vi "垫片有无显示ROI - 副本.vi"(0 "原始图像 IN":T4(plugin-control), 1 "Font, Size & Style":T1={"Desired Font (Application)"=enum."Application Font", "[User-specified Font]"={"Font Name"="", "Size"=100, "Strikeout?"=FALSE, "Italic?"=FALSE, "Underline?"=FALSE, "Outline?"=FALSE, "Shadow?"=FALSE, "Bold?"=TRUE, "Rotation Angle"=0.0}, "Horizontal Alignment"=0, "Vertical Alignment"=0} {"Horizontal Alignment" items=["Left", "Center", "Right"]; "Vertical Alignment" items=["Bottom", "Top", "Baseline"]}, 3 "Center X":i32, 5 "ROI Descriptor":T3 {"Contours"."Type" items=["No Selection", "Point", "Line", "Rectangle", "Oval", "Polygon", "Freehand Region", "Annulus", "Unused2", "Unused3", "Broken Line", "Freehand Line", "Rotated Rectangle"]}, 9 "黑像素阀值判定个数":dbl, 11 "error in (no error)":errorcluster caption="错误输入（无错误）", 12 "黑像个数":dbl, 13 "Center Y":i32) -> (4 "原始图像 OUT":T4(plugin-control), 6 "铜片有/无":bool, 10 "异常":bool, 15 "error out":errorcluster caption="错误输出")   [LabVIEW 2017]
panel:
  out "Annulus":T2 {"End Angle" min=-90.0 max=90.0 step=1.0 format="%.2f"; "Start Angle" min=-90.0 max=90.0 step=1.0 format="%.2f"; "Center X" scale=0.0..1024.0}
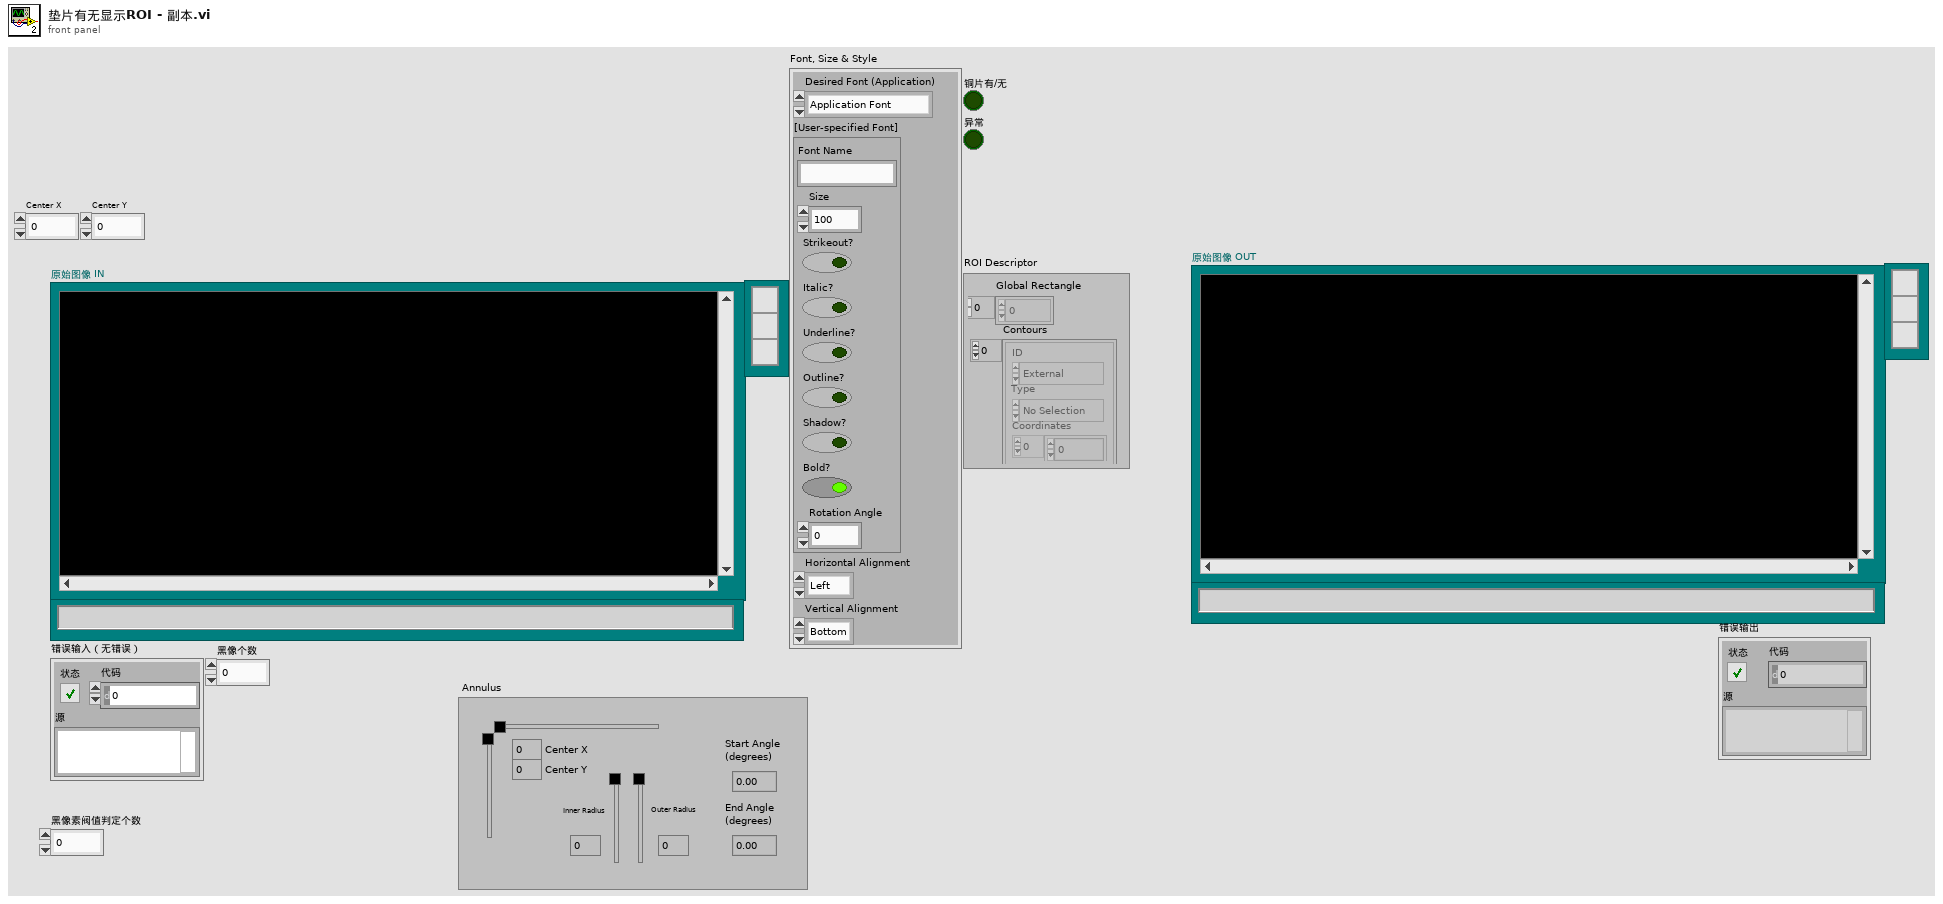
[diagram p1: front panel]
types:
  T1 = cluster{"Desired Font (Application)":enum16{"User-specified Font", "Application Font", "System Font", "Dialog Font"}, "[User-specified Font]":cluster{"Font Name":string, "Size":i16, "Strikeout?":bool, "Italic?":bool, "Underline?":bool, "Outline?":bool, "Shadow?":bool, "Bold?":bool, "Rotation Angle":dbl}, "Horizontal Alignment":i16, "Vertical Alignment":i16}
  T2 = typedef "IMAQ Circle" = cluster{"Center X":i32, "Center Y":i32, "Inner Radius":i32, "Outer Radius":i32, "Start Angle":dbl, "End Angle":dbl}
  T3 = typedef "ROI Descriptor" = cluster{"Global Rectangle":i32[], "Contours":cluster{"ID":enum32{"External", "Internal"}, "Type":u32, "Coordinates":i32[]}[]}
  T4 = typedef "IMAQ Image.ctl" = refnum<image>
  T5 = cluster{"Left":i32, "Top":i32, "rigte":i32, "bottom 3":i32}
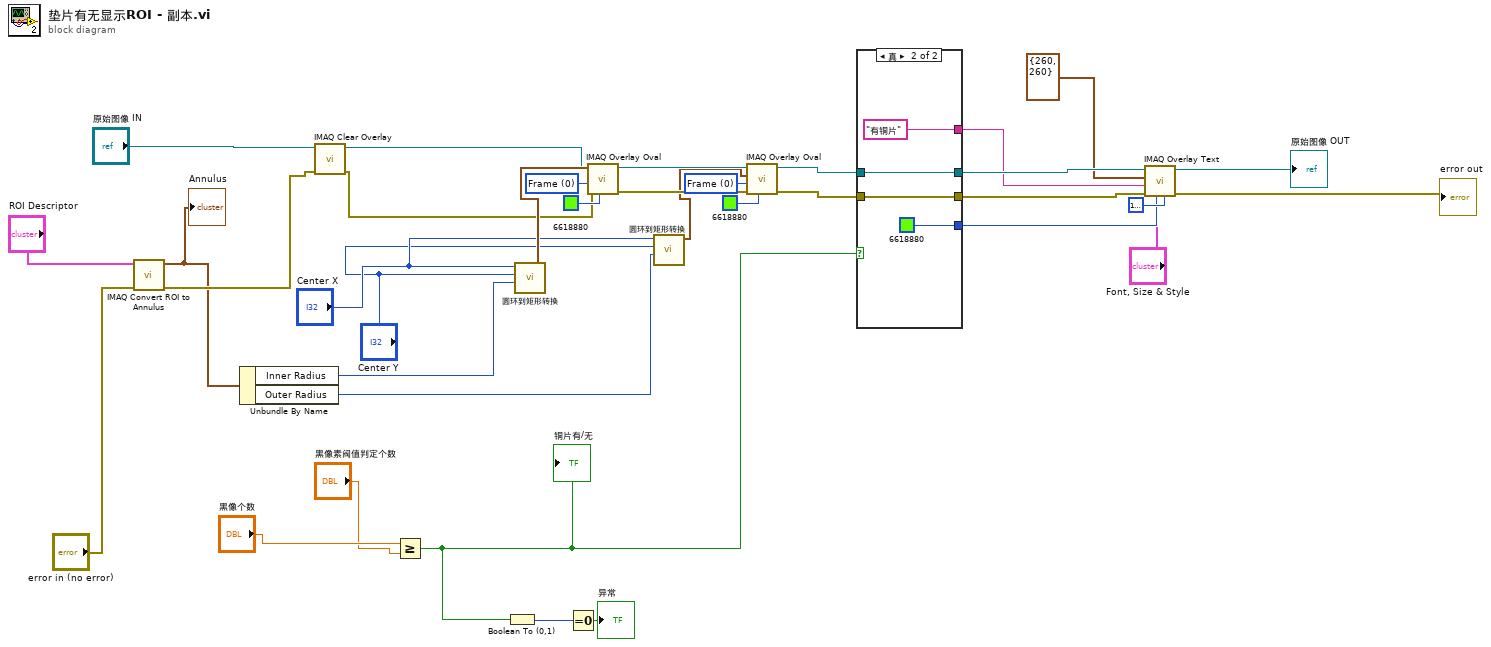
[diagram p0: block diagram]
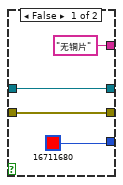
[diagram p2: hidden frame]
diagram:
  w32 = u32 0 items=["Frame", "Fill"] ("Drawing Mode (Frame)")
  w35 = u32 0 items=["Frame", "Fill"] ("Drawing Mode (Frame)")
  n1 = call "IMAQ Convert ROI to Annulus"("error in (no error)"="error in (no error)", "ROI Descriptor"="ROI Descriptor") -> ("error out"=w10:errorcluster, "Annulus"=w2:T2)  [unwired: 7 in]
  "Annulus" <- w2
  n2 = Unbundle By Name(w2) -> ("Inner Radius"=w27:i32, "Outer Radius"=w25:i32)
  n3 = call "IMAQ Clear Overlay"("error in (no error)"=w10, "Image"="原始图像 IN") -> ("error out"=w9:errorcluster, "Image Out"=w11:T4)  [unwired: 8 in]
  n4 = Greater Or Equal?(x="黑像个数", y="黑像素阀值判定个数") -> (x >= y?=w8:bool)
  "铜片有/无" <- w8
  n5 = Boolean To (0,1)(Boolean=w8) -> (0, 1=w7:i16)
  n6 = call "圆环到矩形转换.vi"("Radius"=w27, "CenerY"="Center Y", "CenerX"="Center X") -> ("Bounding Rectangle out"=w28:T5)  [unwired: 8 in]
  n7 = Equal To 0?(x=w7) -> (x = 0?=→"异常":bool)
  n8 = call "IMAQ Overlay Oval"("Color"=u32 6618880, "error in (no error)"=w9, "Drawing Mode (Frame)"=w35, "Bounding Rectangle"=w28, "Image"=w11) -> ("error out"=w33:errorcluster, "Image Out"=w34:T4)  [unwired: 5 in]
  n9 = call "圆环到矩形转换.vi"("Radius"=w25, "CenerY"="Center Y", "CenerX"="Center X") -> ("Bounding Rectangle out"=w26:T5)  [unwired: 8 in]
  n10 = call "IMAQ Overlay Oval"("Color"=u32 6618880, "error in (no error)"=w33, "Drawing Mode (Frame)"=w32, "Bounding Rectangle"=w26, "Image"=w34) -> ("error out"=w21:errorcluster, "Image Out"=w22:T4)  [unwired: 5 in]
  n11 = case shown="真" w8 {
    tunnel: w22 -> [w39 w43]
    tunnel: w21 -> [w38 w42]
    tunnel: [w39 w43] -> w20
    tunnel: [w38 w42] -> w18
    tunnel: ["无铜片" ("String") "有铜片" ("String")] -> w15
    tunnel: [u32 16711680 ("Text Color (black)") u32 6618880 ("Text Color (black)")] -> w13
    frame False {
    }
    frame True {
    }
  }
  n12 = call "IMAQ Overlay Text"("BG Color (Transparent)"=u32 16777216, "Text Color (black)"=w13, "Font, Size & Style"="Font, Size & Style", "error in (no error)"=w18, "String"=w15, "Origin"=cluster{"X":i32, "Y":i32} {"X"=260, "Y"=260}, "Image"=w20) -> ("error out"=→"error out":errorcluster, "Image Out"=→"原始图像 OUT":T4)  [unwired: 3 in]
